vi "Read Subscription Policy ID.vi"(11 "SubscriptionPolicy":T1) -> (2 "Policy ID":string)   [LabVIEW 2020, in "IMediator.lvlib" / "ISubscriptionPolicy.lvclass"]
doc: "读取订阅策略ID"
uses:
  ISubscriptionPolicy.lvclass
  ISubscriptionPolicy Reference.ctl
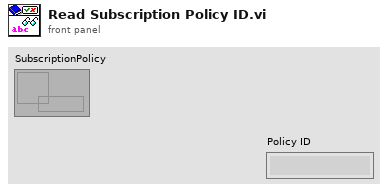
[diagram p1: front panel]
types:
  T1 = typedef "IMediator.lvlib/ISubscriptionPolicy.lvclass/ISubscriptionPolicy Reference.ctl" = refnum<data-value>
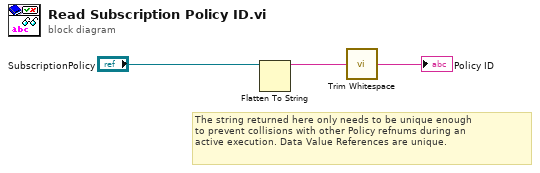
[diagram p0: block diagram]
diagram:
  # "The string returned here only needs to be unique enough\nto prevent collisions with other Policy refnums during an\nactive execution. Data Value References are unique."
  n1 = Flatten To String(anything="SubscriptionPolicy") -> (data string=w2:string)  [unwired: 3 in, 2 out]
  n2 = call <vilib>:"Trim Whitespace.vi"("string"=w2) -> ("trimmed string"=→"Policy ID":string)  [unwired: 1 in]
